vi "set.Field.Value.vi"(8 "error in (no error)":errorcluster, 9 "Value":T1, 10 "FIeld.Name":string="Length", 11 "PitchMessage in":refnum<class "PitchMessage.lvclass">) -> (0 "error out":errorcluster, 3 "PitchMessage out":refnum<class "PitchMessage.lvclass">)   [LabVIEW 2022 SP3, in "PitchMessage.lvclass"]
uses:
  PitchMessage.lvclass
  FieldValue.ctl
  PitchMessage.lvclass/PitchMessage.ctl
panel:
  in  "variant":variant
  out "FieldType":T2(ring)
  out "Length":i32
  in  "Value":i32=34
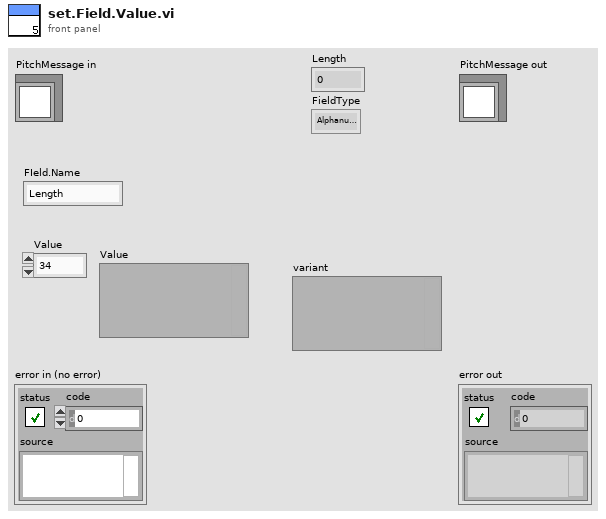
[diagram p1: front panel]
types:
  T1 = typedef "FieldValue.ctl" = variant
  T2 = enum16{"Alphanumeric", "Binary", "BinaryLongPrice", "BinaryShortPrice", "BitField", "PrintableAscii", "Value"}
  T3 = typedef "FieldSpec.ctl" = cluster{"Name":string, "Offset":i32, "Length":i32, "FieldType":enum16{"Alphanumeric", "Binary", "BinaryLongPrice", "BinaryShortPrice", "BitField", "PrintableAscii", "Value"}}
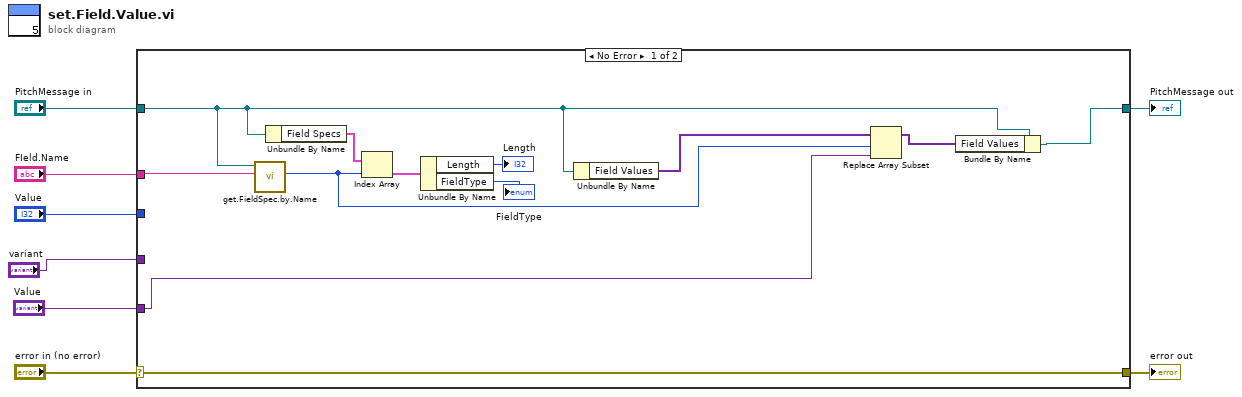
[diagram p0: block diagram]
diagram:
  n1 = case shown="No Error" "error in (no error)" {
    selector: "error in (no error)" -> [w20 w22]
    tunnel: [w20 w22] -> w7
    tunnel: [w10 w21] -> w5
    tunnel: "PitchMessage in" -> [w12 w21]
    tunnel: "FIeld.Name" -> [w15 _]
    tunnel: "Value" -> [_ _]
    tunnel: "Value" -> [w9 _]
    tunnel: "variant" -> [_ _]
    frame No Error {
      n2 = call-dynamic "get.FieldSpec.by.Name.vi"("Field.Name"=w15, "PitchMessage in"=w12) -> ("Index"=w13:i32)  [unwired: 7 in, 2 out]
      n3 = Unbundle By Name(w12) -> ("Field Specs"=w19:T3[])
      n4 = Index Array(array=w19, index=w13) -> (element=w18:T3)
      n5 = Unbundle By Name(w18) -> ("Length"=→"Length":i32, "FieldType"=→"FieldType":T2)
      n6 = Unbundle By Name(w12) -> ("Field Values"=w14:T1[])
      n7 = Replace Array Subset(array=w14, new element=w9, index=w13) -> (w11:T1[])
      n8 = Bundle By Name(cluster=w12, "Field Values"=w11) -> (w10:refnum<class "PitchMessage.lvclass">)
    }
    frame Error {
    }
  }
  "error out" <- w7
  "PitchMessage out" <- w5
